vi "Configure_Graph_Y2.vi"(7 "Execute?":bool, 8 "error in (no error)":errorcluster, 10 "Y2 axis settings":T1={"Y2 axis on/off"=FALSE, "MINIMUM"=0.0, "MAXIMUM"=1.0, "Variable name"="Ig", "LIN or LOG axis"="LIN"} {"MAXIMUM" format="%.9f"; "MINIMUM" format="%.9f"}, 11 "VISA In":refnum<visa-resource-name>) -> (0 "error out":errorcluster, 3 "VISA Out":refnum<visa-resource-name>)   [LabVIEW 2012]
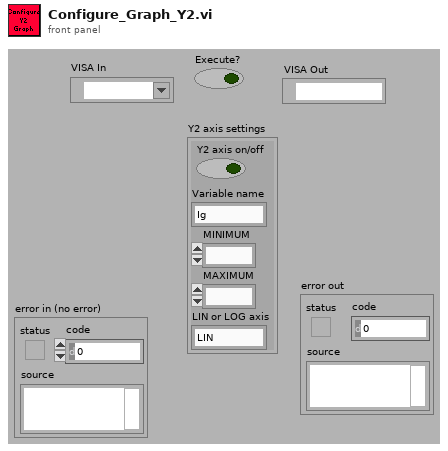
[diagram p1: front panel]
types:
  T1 = cluster{"Y2 axis on/off":bool, "MINIMUM":ext, "MAXIMUM":ext, "Variable name":string, "LIN or LOG axis":string}
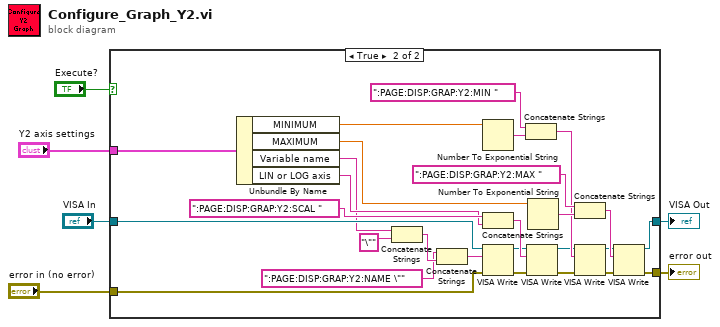
[diagram p0: block diagram]
diagram:
  n1 = case shown="True" "Execute?" {
    tunnel: [w7 w35] -> w6
    tunnel: "error in (no error)" -> [w7 w34]
    tunnel: "VISA In" -> [w8 w15]
    tunnel: [w8 w14] -> w3
    tunnel: "Y2 axis settings" -> [_ w13]
    frame False {
    }
    frame True {
      n2 = Unbundle By Name(w13) -> ("MINIMUM"=w12:ext, "MAXIMUM"=w11:ext, "Variable name"=w9:string, "LIN or LOG axis"=w10:string)
      n3 = Concatenate Strings(w9, "\"" ("string")) -> (w17:string)
      n4 = Concatenate Strings(":PAGE:DISP:GRAP:Y2:NAME \"" ("write buffer"), w17) -> (w19:string)
      n5 = Number To Exponential String(number=w12) -> (E-format string=w29:string)  [unwired: 3 in]
      n6 = Concatenate Strings(":PAGE:DISP:GRAP:Y2:SCAL " ("write buffer"), w10) -> (w27:string)
      n7 = VISA Write(VISA resource name=w15, write buffer=w19, error in (no error)=w34) -> (VISA resource name out=w20:refnum<visa-resource-name>, error out=w23:errorcluster)  [unwired: 1 out]
      n8 = Concatenate Strings(":PAGE:DISP:GRAP:Y2:MIN " ("write buffer"), w29) -> (w30:string)
      n9 = VISA Write(VISA resource name=w20, write buffer=w27, error in (no error)=w23) -> (VISA resource name out=w21:refnum<visa-resource-name>, error out=w24:errorcluster)  [unwired: 1 out]
      n10 = Number To Exponential String(number=w11) -> (E-format string=w31:string)  [unwired: 3 in]
      n11 = Concatenate Strings(":PAGE:DISP:GRAP:Y2:MAX " ("write buffer"), w31) -> (w33:string)
      n12 = VISA Write(VISA resource name=w21, write buffer=w30, error in (no error)=w24) -> (VISA resource name out=w22:refnum<visa-resource-name>, error out=w25:errorcluster)  [unwired: 1 out]
      n13 = VISA Write(VISA resource name=w22, write buffer=w33, error in (no error)=w25) -> (VISA resource name out=w14:refnum<visa-resource-name>, error out=w35:errorcluster)  [unwired: 1 out]
    }
  }
  "error out" <- w6
  "VISA Out" <- w3
